vi "Set CellFormat to DateTime.vi"(8 "error in":errorcluster, 10 "Cell in":refnum<k24>, 11 "SpreadsheetDoc in":refnum<k24>) -> (0 "error out":errorcluster, 2 "Cell out":refnum<k24>, 3 "SpreadsheetDoc out":refnum<k24>)   [LabVIEW 2019, in "Open Xml.lvlib"]
uses:
  Open Xml.lvlib
  D:/git/Open-Xml-LabVIEW/Source/DocumentFormat.OpenXml.dll
  DocumentFormat.OpenXml.dll
  D:/git/Open-Xml-LabVIEW/Source/DocumentFormat.OpenXml.Framework.dll
  DocumentFormat.OpenXml.Framework.dll
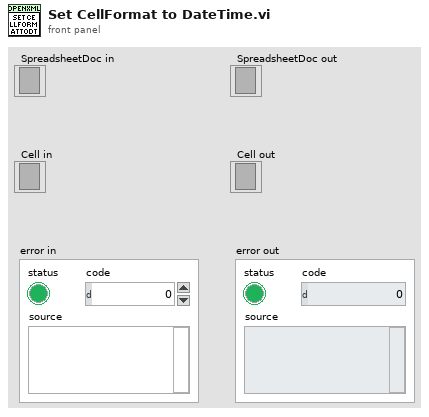
[diagram p1: front panel]
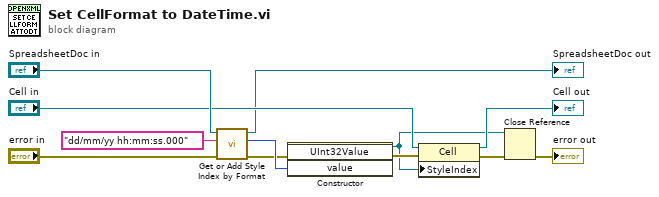
[diagram p0: block diagram]
diagram:
  n1 = call "Get or Add Style Index by Format.vi"("error in"="error in", "Format"="dd/mm/yy hh:mm:ss.000", "SpreadsheetDoc in"="SpreadsheetDoc in") -> ("error out"=w7:errorcluster, "Style Index"=w8:u32, "SpreadsheetDoc out"=→"SpreadsheetDoc out":refnum<k24>)  [unwired: 6 in]
  n2 = constructor class="UInt32Value"(error in=w7, "value"=w8) -> (reference out=w2:refnum<k24>, error out=w6:errorcluster)  [unwired: 2 in, 2 out]
  n3 = property class="Cell"(reference="Cell in", error in=w6, "StyleIndex"=w2) -> (reference out=→"Cell out":refnum<k24>, error out=w11:errorcluster)
  n4 = Close Reference(reference=w2, error in (no error)=w11) -> (error out=→"error out":errorcluster)
